vi "Receive DS Packet.vi"(0 "Recv Socket":refnum<k16>, 5 "Log User Data":bool) -> (2 "New Dashboard Data":bool, 3 "Battery":sgl, 4 "Error Strings":string, 6 "Driver Station":T1, 8 "Robot IP Address":string="10.0.0.2", 10 "Status":T3, 13 "Low Priority User Data":string, 14 "High Priority User Data":string, 15 "Error":T2)   [LabVIEW 2013]
uses:
  DStoPCPacketTypeDef.ctl
panel:
  out "CRC":string
  out "Team ID":u16
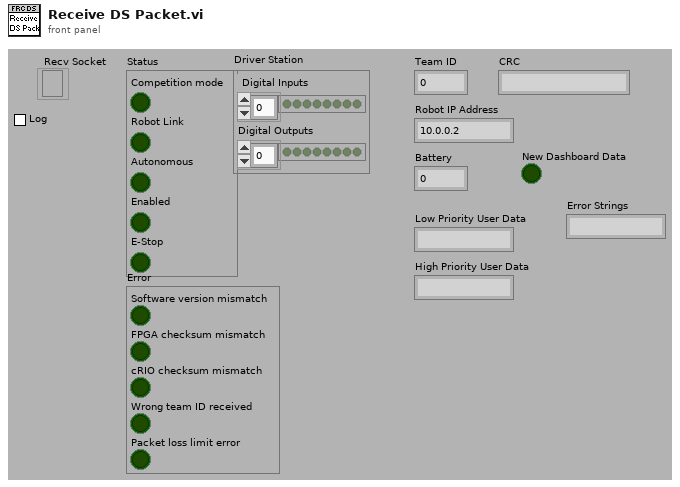
[diagram p1: front panel]
types:
  T1 = cluster{"Digital Inputs":bool[], "Digital Outputs":bool[]}
  T2 = cluster{"Software version mismatch":bool, "FPGA checksum mismatch":bool, "cRIO checksum mismatch":bool, "Wrong team ID received":bool, "Packet loss limit error":bool}
  T3 = cluster{"Competition mode":bool, "Robot Link":bool, "Autonomous":bool, "Enabled":bool, "E-Stop":bool}
  T4 = typedef "DStoPCPacketTypeDef.ctl" = cluster{"Packet Index":u16, "Digital Inputs":u8, "Digital Out":u8, "Battery":u16, "Status":u8, "Error":u8, "Team ID":u16, "VersionMonth1":u8, "VersionMonth2":u8, "VersionDay1":u8, "VersionDay2":u8, "VersionYear1":u8, "VersionYear2":u8, "Revision1":u8, "Revision2":u8, "UnusedBuffer":u32, "UnusedBuffer 2":u16, "Reply Packet #":u16}
  T5 = cluster{"Boolean array":bool[], "Boolean array":bool[]}
  T6 = cluster{"Boolean array[0]":bool, "Boolean array[1]":bool, "Boolean array[2]":bool, "Boolean array[3]":bool, "Boolean array[4]":bool, "Boolean array[5]":bool, "Boolean array[6]":bool, "Boolean array[7]":bool}
  T7 = cluster{"Boolean array[0]":bool, "Boolean array[1]":bool, "Boolean array[4]":bool, "Boolean array[5]":bool, bool}
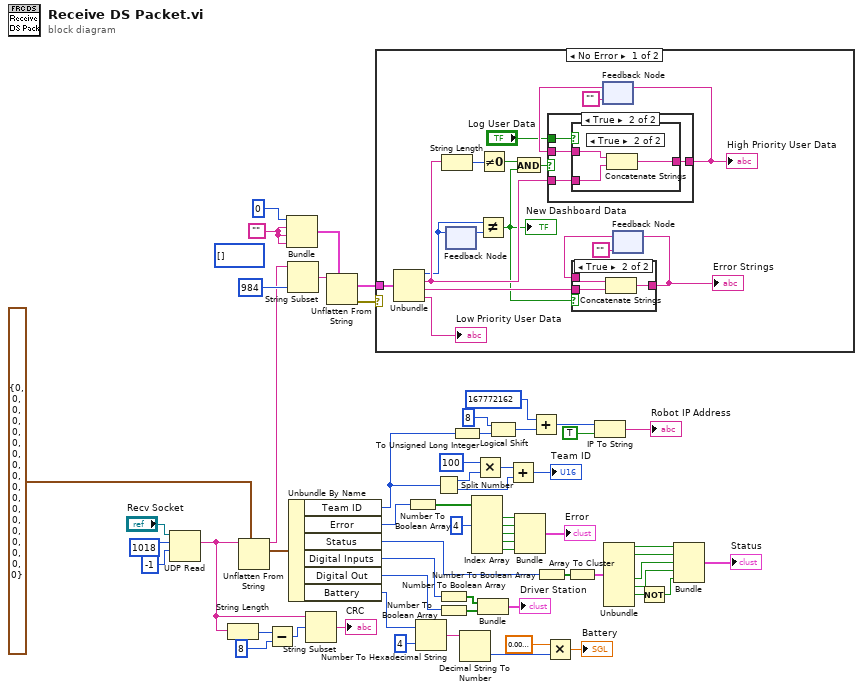
[diagram p0: block diagram]
diagram:
  (unwired) u8[] []
  w1 = ""
  n1 = UDP Read(connection ID="Recv Socket", max size (548)=1018 ("bytes to read"), timeout ms (25000)=-1) -> (data out=w21:string)  [unwired: 1 in, 4 out]
  n2 = String Length(string=w21) -> (length=w33:i32)
  n3 = Unflatten From String(type=T4 {"Packet Index"=0, "Digital Inputs"=0, "Digital Out"=0, "Battery"=0, "Status"=0, "Error"=0, "Team ID"=0, "VersionMonth1"=0, "VersionMonth2"=0, "VersionDay1"=0, "VersionDay2"=0, "VersionYear1"=0, "VersionYear2"=0, "Revision1"=0, "Revision2"=0, "UnusedBuffer"=0, "UnusedBuffer 2"=0, "Reply Packet #"=0} ("Cluster"), binary string=w21) -> (rest of the binary string=w34:string, value=w61:T4)  [unwired: 1 in, 3 out]
  n4 = Subtract(x=w33, y=8) -> (x-y=w31:i32)
  n5 = Bundle(u8 0, w1, w1, w1) -> (w5:cluster{u8, string, string, string})  [unwired: 1 out]
  n6 = String Subset(string=w34, length (rest)=984 ("length (rest)")) -> (substring=w10:string)  [unwired: 1 out]
  n7 = Unbundle By Name(w61) -> ("Team ID"=w39:u16, "Error"=w52:u8, "Status"=w60:u8, "Digital Inputs"=w9:u8, "Digital Out"=w8:u8, "Battery"=w28:u16)
  n8 = String Subset(string=w21, offset (0)=w31) -> (substring=→"CRC":string)  [unwired: 1 out]
  n9 = Unflatten From String(type=w5, binary string=w10) -> (value=w3:cluster{u8, string, string, string}, error out=w2:errorcluster)  [unwired: 1 in, 3 out]
  n10 = case shown="No Error" w2 {
    tunnel: w3 -> [w75 _]
    frame No Error {
      n11 = Unbundle(w75) -> (w66:u8, w67:string, w73:string, →"Low Priority User Data":string)
      n12 = String Length(string=w67) -> (length=w68:i32)
      n13 = feedback-in #1(w66) -> ()
      n14 = feedback #1() -> (w65:u8)  [unwired: 1 out]
      n15 = Not Equal?(x=w66, y=w65) -> (x != y?=w64:bool)
      "New Dashboard Data" <- w64
      n16 = Not Equal To 0?(x=w68) -> (x != 0?=w69:bool)
      n17 = And(x=w69, y=w64) -> (x .and. y?=w70:bool)
      n18 = feedback #2("") -> (w76:string)
      n19 = case shown="True" w70 {
        tunnel: w67 -> [_ w87]
        tunnel: [w83 w86] -> w62
        tunnel: w76 -> [w83 w85]
        tunnel: "Log User Data" -> [_ w84]
        frame False {
        }
        frame True {
          n20 = case shown="True" w84 {
            tunnel: w87 -> [w88 w91]
            tunnel: [w88 w90] -> w86
            tunnel: w85 -> [_ w89]
            frame False {
            }
            frame True {
              n21 = Concatenate Strings(w89, w91) -> (w90:string)
            }
          }
        }
      }
      "High Priority User Data" <- w62
      n22 = feedback-in #2(w62) -> ()
      n23 = feedback #3("") -> (w78:string)
      n24 = case shown="True" w64 {
        tunnel: [w79 w82] -> w63
        tunnel: w78 -> [w79 w81]
        tunnel: w73 -> [_ w80]
        frame False {
        }
        frame True {
          n25 = Concatenate Strings(w81, w80) -> (w82:string)
        }
      }
      "Error Strings" <- w63
      n26 = feedback-in #3(w63) -> ()
    }
    frame Error {
    }
  }
  n27 = Number To Boolean Array(number=w52) -> (Boolean array=w17:bool[])
  n28 = Number To Hexadecimal String(1:i16 4 ("width (-)"), 2:w28) -> (0:w27:string)
  n29 = Split Number(x=w39) -> (hi(x)=w49:u8, lo(x)=w46:u8)
  n30 = Number To Boolean Array(number=w9) -> (Boolean array=w6:bool[])
  n31 = Number To Boolean Array(number=w8) -> (Boolean array=w7:bool[])
  n32 = To Unsigned Long Integer(number=w39) -> (unsigned 32bit integer=w43:u32)
  n33 = Decimal String To Number(string=w27) -> (number=w25:i32)  [unwired: 3 out]
  n34 = Index Array(array=w17, index #2=4 ("index")) -> (element #1=w11:bool, element #2=w12:bool, element #3=w13:bool, element #4=w14:bool, element #5=w15:bool)  [unwired: 4 in]
  n35 = Multiply(x=u16 100, y=w49) -> (x*y=w47:u16)
  n36 = Bundle("Boolean array"=w6, "Boolean array"=w7) -> (→"Driver Station":T5)  [unwired: 1 out]
  n37 = Logical Shift(y=i8 8, x=w43) -> (x << y=w41:u32)
  n38 = Add(x=w47, y=w46) -> (x+y=→"Team ID":u16)
  n39 = Bundle(w11, w12, w13, w14, w15) -> (→"Error":cluster{bool, bool, bool, bool, bool})  [unwired: 1 out]
  n40 = Add(x=u32 167772162 ("address"), y=w41) -> (x+y=w37:u32)
  n41 = Number To Boolean Array(number=w60) -> (Boolean array=w59:bool[])
  n42 = Multiply(x=sgl 0.01, y=w25) -> (x*y=→"Battery":sgl)
  n43 = Array To Cluster(array=w59) -> (cluster=w57:T6)
  n44 = IP To String(1:TRUE ("dot notation? (F)"), 2:w37) -> (0:→"Robot IP Address":string)
  n45 = Unbundle(w57) -> ("Boolean array[0]"=w56:bool, "Boolean array[1]"=w55:bool, "Boolean array[4]"=w54:bool, "Boolean array[5]"=w53:bool, "Boolean array[6]"=w51:bool)  [unwired: 3 out]
  n46 = Not(x=w51) -> (.not. x?=w50:bool)
  n47 = Bundle("Boolean array[0]"=w56, "Boolean array[1]"=w55, "Boolean array[4]"=w54, "Boolean array[5]"=w53, w50) -> (→"Status":T7)  [unwired: 1 out]
